vi "buffer array clust.vi"(0 "Array":dbl[](array[numeric]), 1 "History length":i32, 2 "Log":T1=enum."TimeStamp", 10 "Start channel":i32) -> ()   [LabVIEW 2018]
uses:
  history_array_type.ctl
  CAEN globals.vi
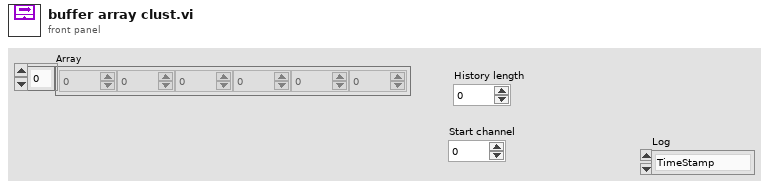
[diagram p1: front panel]
types:
  T1 = typedef "history_array_type.ctl" = enum16{"Vmon", "Vset", "Imon", "Iset", "TimeStamp"}
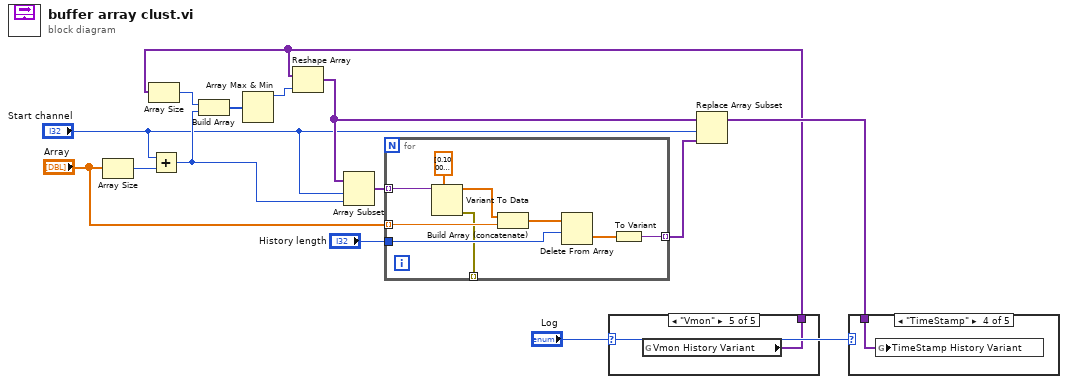
[diagram p0: block diagram]
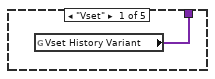
[diagram p2: hidden frame]
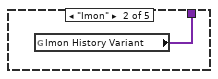
[diagram p3: hidden frame]
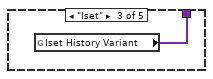
[diagram p4: hidden frame]
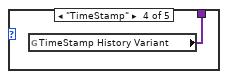
[diagram p5: hidden frame]
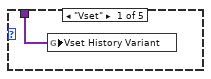
[diagram p6: hidden frame]
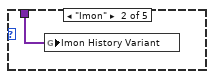
[diagram p7: hidden frame]
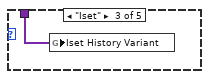
[diagram p8: hidden frame]
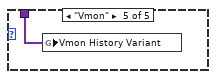
[diagram p9: hidden frame]
diagram:
  n1 = Array Size(array="Array") -> (size(s)=w12:i32)
  n2 = Add(x="Start channel", y=w12) -> (x+y=w9:i32)
  n3 = case shown="\"Vmon\"" "Log" {
    tunnel: [w15 w16 w17 w18 w19] -> w1
    frame "Vset" {
      n4 = global read "CAEN globals.vi" "Vset History Variant"() -> (w15:variant[])
    }
    frame "Imon" {
      n5 = global read "CAEN globals.vi" "Imon History Variant"() -> (w16:variant[])
    }
    frame "Iset" {
      n6 = global read "CAEN globals.vi" "Iset History Variant"() -> (w17:variant[])
    }
    frame "TimeStamp" {
      n7 = global read "CAEN globals.vi" "TimeStamp History Variant"() -> (w18:variant[])
    }
    frame "Vmon" {
      n8 = global read "CAEN globals.vi" "Vmon History Variant"() -> (w19:variant[])
    }
  }
  n9 = Array Size(array=w1) -> (size(s)=w11:i32)
  n10 = Build Array(w11, w9) -> (w13:i32[])
  n11 = Array Max & Min(array=w13) -> (max value=w14:i32)  [unwired: 3 out]
  n12 = Reshape Array(w1, w14) -> (w10:variant[])
  n13 = Array Subset(array=w10, index="Start channel", length=w9) -> (w8:variant[])
  n14 = for {
    tunnel: w8 -> [w28] mode=indexing
    tunnel: "Array" -> [w26] mode=indexing
    tunnel: [w24] -> w7 mode=indexing
    tunnel: "History length" -> [w22]
    tunnel: [w20] -> _ mode=indexing
    n15 = Variant To Data(type=dbl[] [0.10000000000000009, 0.20000000000000018, 1.2999999999999998] ("Value"), Variant=w28) -> (data=w25:dbl[], error out=w20:errorcluster)  [unwired: 1 in]
    n16 = Build Array (concatenate)(w25, w26) -> (w23:dbl[])
    n17 = Delete From Array(array=w23, length=w22) -> (deleted portion=w21:dbl[])  [unwired: 1 in, 1 out]
    n18 = To Variant(anything=w21) -> (Variant=w24:variant)
  }
  n19 = Replace Array Subset(array=w10, new element=w7, index="Start channel") -> (w2:variant[])
  n20 = case shown="\"TimeStamp\"" "Log" {
    tunnel: w2 -> [w29 w30 w31 w32 w33]
    frame "Vset" {
      n21 = global write "CAEN globals.vi" "Vset History Variant"(w29) -> ()
    }
    frame "Imon" {
      n22 = global write "CAEN globals.vi" "Imon History Variant"(w30) -> ()
    }
    frame "Iset" {
      n23 = global write "CAEN globals.vi" "Iset History Variant"(w31) -> ()
    }
    frame "TimeStamp" {
      n24 = global write "CAEN globals.vi" "TimeStamp History Variant"(w32) -> ()
    }
    frame "Vmon" {
      n25 = global write "CAEN globals.vi" "Vmon History Variant"(w33) -> ()
    }
  }
